vi "Read Terminals.vi"(8 "error in":errorcluster, 11 "channel ref in":refnum<k20>) -> (0 "error out":errorcluster, 1 "terminal names":string[](array[string]), 2 "terminal addresses":T1[](array[typedef]), 3 "channel ref out":refnum<k20>)   [LabVIEW 2020, in "AIM MIL-STD 1553 Import.lvlib"]
uses:
  AIM MIL-STD 1553 Import.lvlib
  Constants.vi
  959ec5e7-4734-4cf0-9432-93ed95d58c03.vi
  5dfed85f-e5be-47f3-b024-20b595401d52.vi
  Shared/Address.ctl
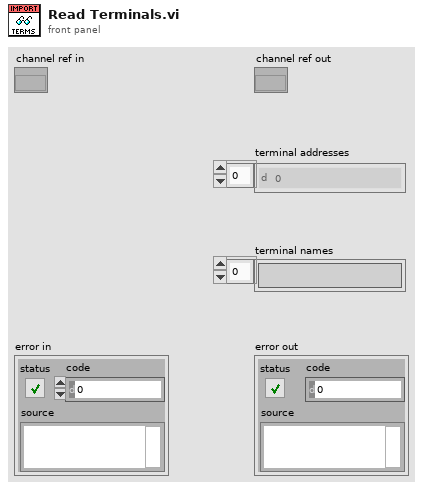
[diagram p1: front panel]
types:
  T1 = typedef "Address.ctl" = u16
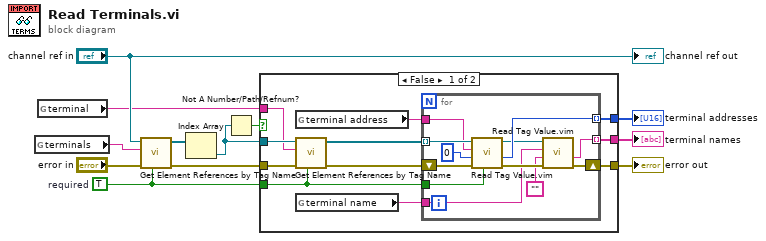
[diagram p0: block diagram]
diagram:
  w4 = TRUE  # required
  n1 = global read "Constants.vi" "terminals"() -> (w3:string)
  n2 = global read "Constants.vi" "terminal"() -> (w2:string)
  n3 = call "Get Element References by Tag Name.vi"("required (F)"=w4, "error in"="error in", "tag name"=w3, "node in"="channel ref in") -> ("error out"=w7:errorcluster, "array of elements"=w8:refnum<k20>[])  [unwired: 6 in]
  n4 = Index Array(array=w8) -> (element=w5:refnum<k20>)  [unwired: 1 in]
  n5 = Not A Number/Path/Refnum?(number/path/refnum=w5) -> (NaN/Path/Refnum?=w6:bool)
  n6 = case shown="False" w6 {
    tunnel: [w23 w36] -> w12
    tunnel: [w22 _] -> w9
    tunnel: w5 -> [w21 _]
    tunnel: w7 -> [w20 w36]
    tunnel: w4 -> [w15 _]
    tunnel: w2 -> [w19 _]
    tunnel: [w13 _] -> w1
    frame False {
      n7 = global read "Constants.vi" "terminal address"() -> (w16:string)
      n8 = call "Get Element References by Tag Name.vi"("required (F)"=w15, "error in"=w20, "tag name"=w19, "node in"=w21) -> ("error out"=w17:errorcluster, "array of elements"=w18:refnum<k20>[])  [unwired: 6 in]
      n9 = global read "Constants.vi" "terminal name"() -> (w14:string)
      n10 = for {
        shift-right: [w27] -> w23
        shift-left: w17 -> [w34]
        tunnel: [w30] -> w22 mode=indexing
        tunnel: w18 -> [w35] mode=indexing
        tunnel: w16 -> [w33]
        tunnel: w15 -> [w32]
        tunnel: w14 -> [w26]
        tunnel: [w24] -> w13 mode=indexing
        n11 = call "Read Tag Value.vim"("required (F)"=w32, "error in"=w34, "default"=u16 0, "tag name"=w33, "node in"=w35) -> ("error out"=w28:errorcluster, "value"=w30:u16, "node out"=w29:refnum<k20>)  [unwired: 4 in]
        n12 = call "Read Tag Value.vim"("error in"=w28, "default"="", "tag name"=w26, "node in"=w29) -> ("error out"=w27:errorcluster, "value"=w24:string)  [unwired: 5 in, 1 out]
      }
    }
    frame True {
    }
  }
  "error out" <- w12
  "terminal addresses" <- w9
  "terminal names" <- w1
  "channel ref out" <- "channel ref in"
